vi "空载计算.vi"(10 "扭矩数组":dbl[](array[numeric])) -> (1 "空载扭差":dbl format="%#.2f", 2 "空载平均扭矩":dbl format="%#.2f", 3 "空载峰值扭矩":dbl format="%#.2f")   [LabVIEW 2013]
panel:
  out "第一个子数组":dbl[](array[numeric])
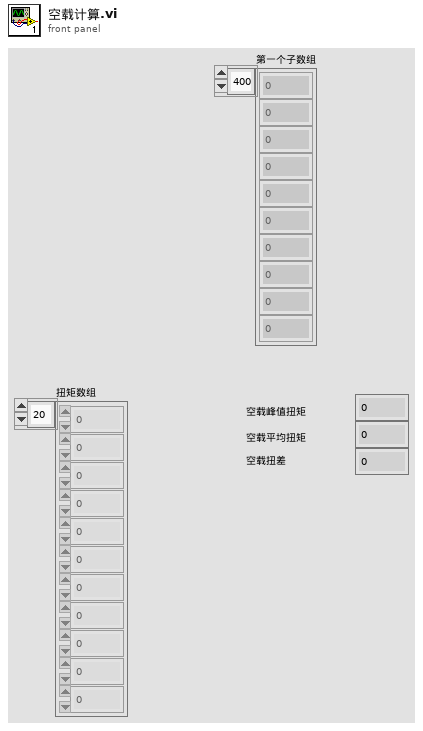
[diagram p1: front panel]
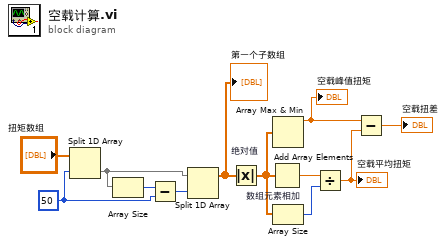
[diagram p0: block diagram]
diagram:
  w2 = 50 ("索引")
  n1 = Split 1D Array(array="扭矩数组", index=w2) -> (second subarray=w4:dbl[])  [unwired: 1 out]
  n2 = Array Size(array=w4) -> (size(s)=w3:i32)
  n3 = Subtract(x=w3, y=w2) -> (x-y=w1:i32)
  n4 = Split 1D Array(array=w4, index=w1) -> (first subarray=w8:dbl[])  [unwired: 1 out]
  "第一个子数组" <- w8
  n5 = Absolute Value "绝对值"(x=w8) -> (abs(x)=w10:dbl[])
  n6 = Add Array Elements "数组元素相加"(numeric array=w10) -> (sum=w11:dbl)
  n7 = Array Max & Min(array=w10) -> (max value=w7:dbl)  [unwired: 3 out]
  "空载峰值扭矩" <- w7
  n8 = Array Size(array=w10) -> (size(s)=w9:i32)
  n9 = Divide(x=w11, y=w9) -> (x/y=w6:dbl)
  "空载平均扭矩" <- w6
  n10 = Subtract(x=w7, y=w6) -> (x-y=→"空载扭差":dbl)
